vi "ArmFF_Calculate.vi"(8 "AccelRadPerSecSquared":dbl, 9 "VelocityRadiansPerSec":dbl, 10 "PositionRadians":dbl, 11 "in ARM_FF":T1 {"kCos" format="%13.5p"; "Ka" format="%13.5p"; "Kv" format="%13.5p"; "Ks" format="%13.5p"}) -> (3 "FeedForward":dbl)   [LabVIEW 2019, in "Trajectory_Library.lvlib"]
doc: "Calculates the feedforward from the gains and setpoints.\n\nInputs: \n - ArmFF -- The ArmFF data cluster\n - positionRadians -- The position (angle) setpoint.\n - velocityRadPerSec -- The velocity setpoint.\n - accelRadPerSecSquared -- The acceleration setpoint.\n\nOutputs:\n - feedForward -- The computed feedforward."
uses:
  Trajectory_Library.lvlib
  TypeDef/ARM_FF.ctl
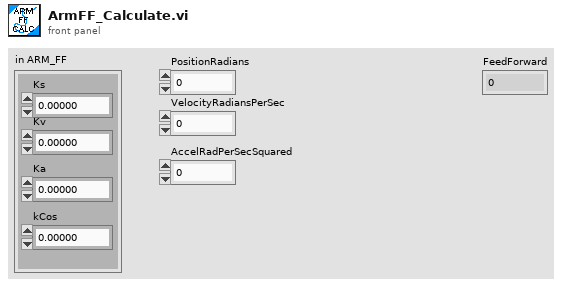
[diagram p1: front panel]
types:
  T1 = typedef "Trajectory_Library.lvlib/ARM_FF.ctl" = cluster{"Ks":dbl, "Kv":dbl, "Ka":dbl, "kCos":dbl}
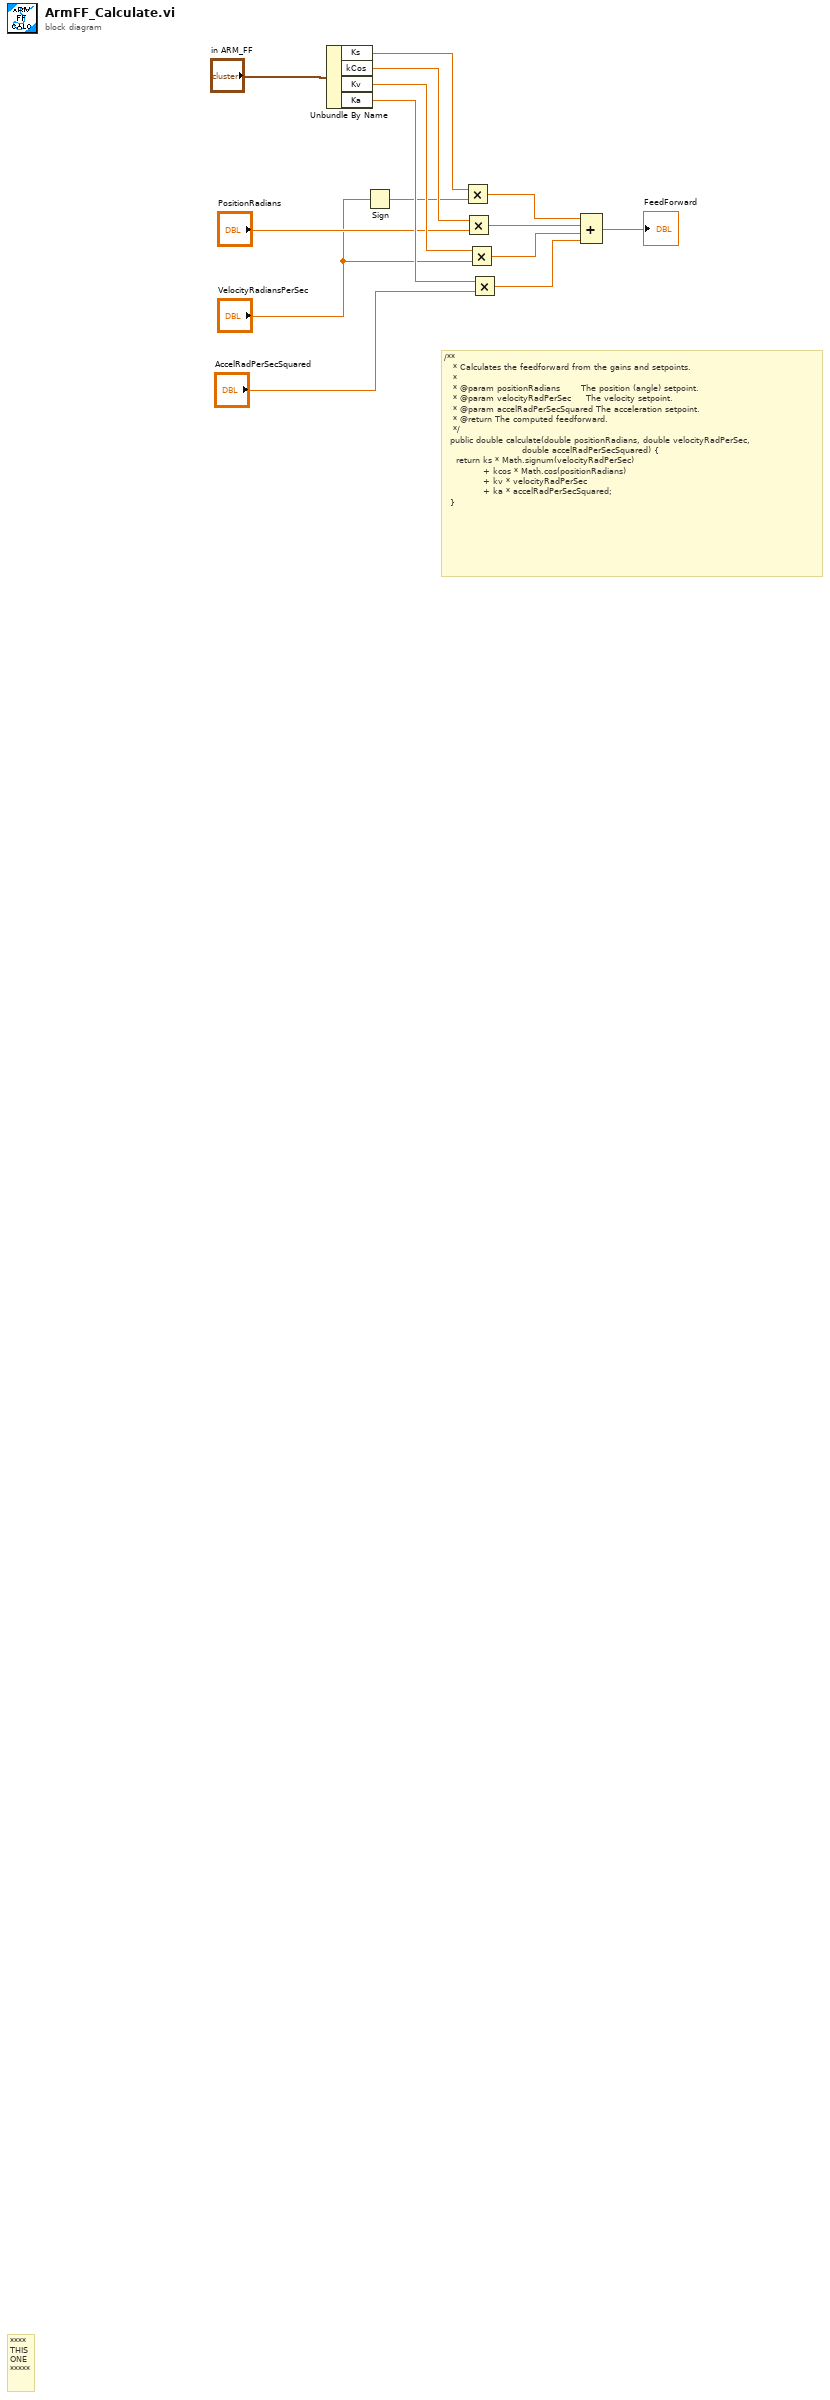
[diagram p0: block diagram]
diagram:
  # "/**\n   * Calculates the feedforward from the gains and setpoints.\n   *\n   * @param positionRadians       The position (angle) setpoint.\n   * @param velocityRadPerSec     The velocity setpoint.\n   * @param accelRadPerSecSquared The acceleration setpoint.\n   * @return The computed feedforward.\n   */\n  public double calculate(double positionRadians, double velocityRadPerSec,\n                          double accelRadPerSecSquared) {\n    return ks * Math.signum(velocityRadPerSec) \n             + kcos * Math.cos(positionRadians)\n             + kv * velocityRadPerSec\n             + ka * accelRadPerSecSquared;\n  }"
  # "****\nTHIS\nONE\n*****"
  n1 = Unbundle By Name("in ARM_FF") -> ("Ks"=w8:dbl, "kCos"=w7:dbl, "Kv"=w6:dbl, "Ka"=w5:dbl)
  n2 = Sign(1:"VelocityRadiansPerSec") -> (0:w4:dbl)
  n3 = Multiply(x=w8, y=w4) -> (x*y=w12:dbl)
  n4 = Multiply(x=w7, y="PositionRadians") -> (x*y=w11:dbl)
  n5 = Multiply(x=w6, y="VelocityRadiansPerSec") -> (x*y=w10:dbl)
  n6 = Multiply(x=w5, y="AccelRadPerSecSquared") -> (x*y=w9:dbl)
  n7 = Compound Arithmetic op=ADD(w12, w11, w10, w9) -> (→"FeedForward":dbl)
